vi "GetState.vi"(11 "Pump_1AI_1DO_2DI in":refnum<class "Valve_2DO_2DI.lvclass">) -> (2 "valveState":T1=enum."Closed")   [LabVIEW 2019, in "Valve_2DO_2DI.lvclass"]
uses:
  Valve_2DO_2DI.lvclass
  FPGA/TypeDef/valveState.ctl
  Valve_2DO_2DI.lvclass/Valve_2DO_2DI.ctl
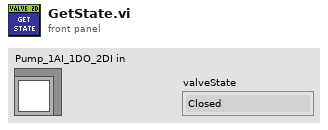
[diagram p1: front panel]
types:
  T1 = typedef "valveState.ctl" = enum16{"Unknown", "Closed", "Opening", "Opened", "Closing"}
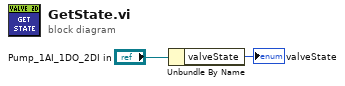
[diagram p0: block diagram]
diagram:
  n1 = Unbundle By Name("Pump_1AI_1DO_2DI in") -> ("valveState"=→"valveState":T1)
